vi "variant2Attributes.vi"(0 "HGV_PVBase":refnum<class "HGF_SVSubscriber.lvclass">, 2 "rawData":variant, 3 "typeDescriptor":string, 5 "error in (no error)":errorcluster) -> (14 "HGV_PVBase":refnum<class "HGF_SVSubscriber.lvclass">, 15 "no link":bool, 16 "Parameter":variant, 17 "typeDescriptor":string, 19 "error out":errorcluster)   [LabVIEW 2012, in "HGF_SV.lvlib" / "HGF_SVSubscriber.lvclass"]
doc: "Convert raw data value of variant to variant attributes Pn, n=0,1,2,..."
uses:
  HGF_SVSubscriber.lvclass
  HGF_BaseClasses/HGF_PVSubscriber/HGF_PVSubscriber.lvclass
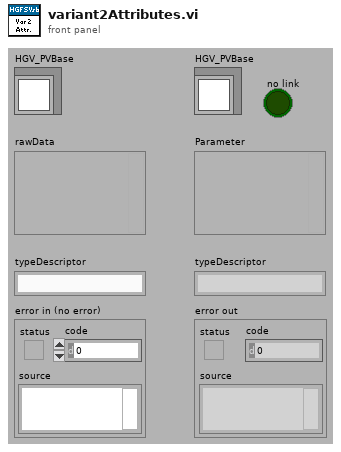
[diagram p1: front panel]
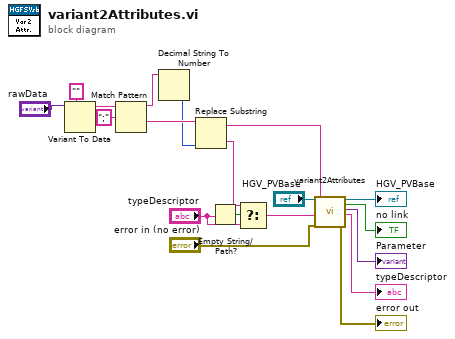
[diagram p0: block diagram]
diagram:
  n1 = Variant To Data(type="" ("typeDescriptor 2"), Variant="rawData") -> (data=w7:string)  [unwired: 1 in, 1 out]
  n2 = Match Pattern(string=w7, regular expression=";") -> (before substring=w5:string, after substring=w4:string)  [unwired: 3 out]
  n3 = Decimal String To Number(string=w5) -> (number=w3:i32)  [unwired: 3 out]
  n4 = Replace Substring(2:w3, 5:w4) -> (0:w2:string, 1:w1:string)  [unwired: 2 out]
  n5 = Empty String/Path?(string/path="typeDescriptor") -> (empty?=w10:bool)
  n6 = Select(t=w2, s=w10, f="typeDescriptor") -> (s? t:f=w12:string)
  n7 = call-parent "variant2Attributes.vi"("HGV_PVBase"="HGV_PVBase", "rawData"=w1, "typeDescriptor"=w12, "error in (no error)"="error in (no error)") -> ("HGV_PVBase"=→"HGV_PVBase":refnum<class "HGF_SVSubscriber.lvclass">, "no link"=→"no link":bool, "Parameter"=→"Parameter":variant, "typeDescriptor"=→"typeDescriptor":string, "error out"=→"error out":errorcluster)  [unwired: 11 out]
